vi "uTTA_FindIllegalCharacters.vi"() -> ()   [LabVIEW 2021]
panel:
  out "String":string
  out "Addresses":u64[](array[numeric]) format="0x%x"
  in  "File Path":path
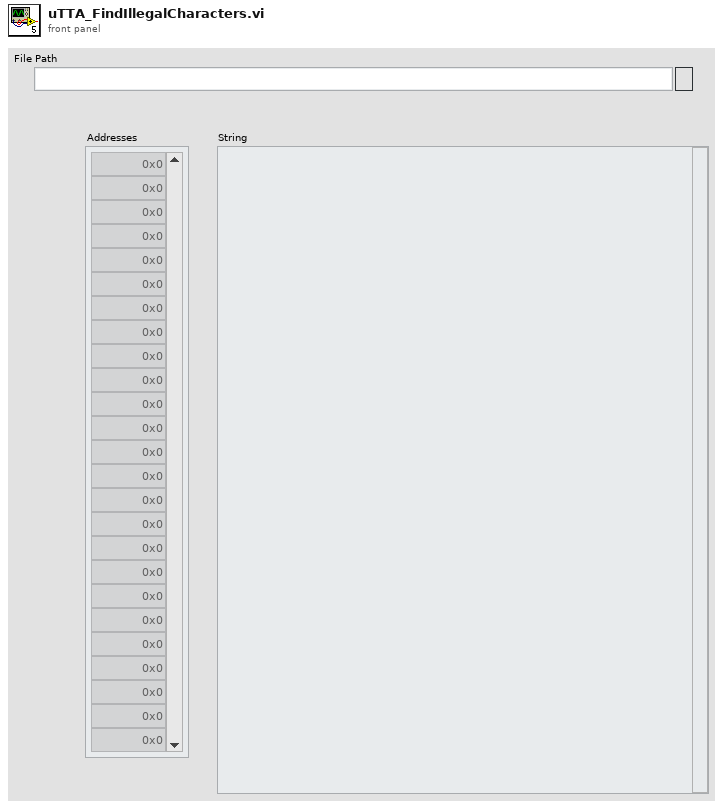
[diagram p1: front panel]
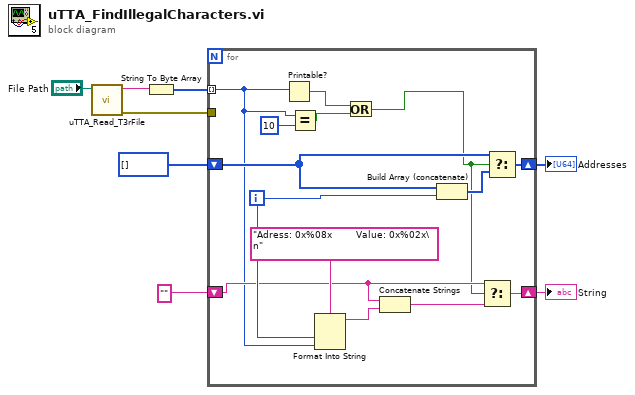
[diagram p0: block diagram]
diagram:
  n1 = call "uTTA_Read_T3rFile.vi"("File Path"="File Path") -> ("error out"=w5:errorcluster, "T3R-File"=w7:string)  [unwired: 8 in, 1 out]
  n2 = String To Byte Array(string=w7) -> (unsigned byte array=w6:u8[])
  n3 = for {
    tunnel: w6 -> [w13] mode=indexing
    tunnel: w5 -> [_]
    shift-right: [w19] -> w1
    shift-left: "" -> [w16]
    shift-right: [w21] -> w2
    shift-left: u64[] [] -> [w20]
    i -> [w18]
    n4 = Printable?(1:w13) -> (0:w10:bool)
    n5 = Equal?(x=w13, y=u8 10) -> (x = y?=w11:bool)
    n6 = Format Into String(format string="Adress: 0x%08x        Value: 0x%02x\n", w18, w13) -> (resulting string=w15:string)  [unwired: 2 in, 1 out]
    n7 = Or(x=w10, y=w11) -> (x .or. y?=w9:bool)
    n8 = Concatenate Strings(w16, w15) -> (w14:string)
    n9 = Build Array (concatenate)(w20, w18) -> (w22:u64[])
    n10 = Select(t=w16, s=w9, f=w14) -> (s? t:f=w19:string)
    n11 = Select(t=w20, s=w9, f=w22) -> (s? t:f=w21:u64[])
  }
  "Addresses" <- w2
  "String" <- w1
